vi "Export Subpanels.vi"() -> (0 "Range":refnum<vi>, 1 "Reader Setup":refnum<vi>, 2 "Scanner Setup":refnum<vi>, 3 "FileIO Setup":refnum<vi>)   [LabVIEW 2012, in "Scan Driver.lvclass"]
uses:
  Scan Driver.lvclass
  Setup.vi
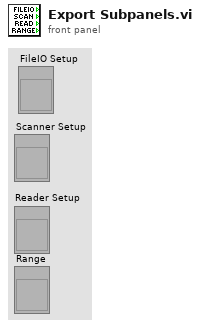
[diagram p1: front panel]
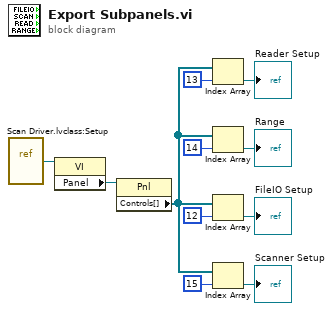
[diagram p0: block diagram]
diagram:
  n1 = vi-ref "Scan Driver.lvclass:Setup.vi"() -> (w11:refnum<vi>)
  n2 = property class="VI"(reference=w11) -> ("Panel"=w10:refnum<vi>)  [unwired: 1 in, 2 out]
  n3 = property class="Pnl"(reference=w10) -> ("Controls[]"=w7:refnum<vi>[])  [unwired: 1 in, 2 out]
  n4 = Index Array(array=w7, index=13) -> (element=→"Reader Setup":refnum<vi>)
  n5 = Index Array(array=w7, index=14) -> (element=→"Range":refnum<vi>)
  n6 = Index Array(array=w7, index=12) -> (element=→"FileIO Setup":refnum<vi>)
  n7 = Index Array(array=w7, index=15) -> (element=→"Scanner Setup":refnum<vi>)
